vi "ge_HideCellCtrls.vi"(8 "error IO":errorcluster, 11 "FP Ctrl":T1) -> (0 "error out":errorcluster)   [LabVIEW 2018]
uses:
  Custom Ctrls/ge_FPCtrlRefLabel.ctl
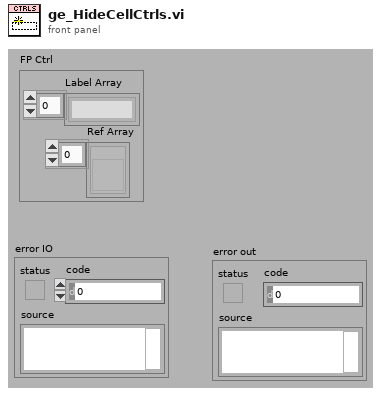
[diagram p1: front panel]
types:
  T1 = typedef "ge_FPCtrlRefLabel.ctl" = cluster{"Label Array":string[], "Ref Array":refnum<vi>[]}
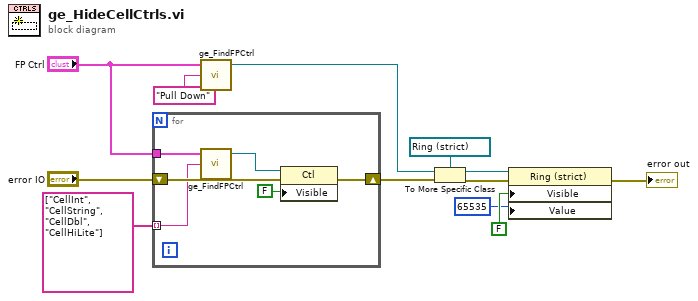
[diagram p0: block diagram]
diagram:
  n1 = for {
    shift-right: [w16] -> w8
    shift-left: "error IO" -> [w18]
    tunnel: string[] ["CellInt", "CellString", "CellDbl", "CellHiLite"] -> [w15] mode=indexing
    tunnel: "FP Ctrl" -> [w14]
    n2 = call "ge_FindFPCtrl.vi"("Ctrl Name"=w15, "FP Ctrl"=w14) -> ("Ctrl Ref"=w13:refnum<vi>)  [unwired: 3 in]
    n3 = property on="Property Node" class="Ctl"(reference=w13, error in=w18, "Visible"=FALSE) -> (error out=w16:errorcluster)  [unwired: 1 out]
  }
  n4 = call "ge_FindFPCtrl.vi"("Ctrl Name"="Pull Down" ("Name"), "FP Ctrl"="FP Ctrl") -> ("Ctrl Ref"=w5:refnum<vi>)  [unwired: 3 in]
  n5 = To More Specific Class(target class=refnum<vi> refnum ("reference"), reference=w5, error in=w8) -> (specific class reference=w1:refnum<vi>, error out=w4:errorcluster)
  n6 = property on="Property Node" class="Ring (strict)"(reference=w1, error in=w4, "Visible"=FALSE, "Value"=u16 65535) -> (error out=→"error out":errorcluster)  [unwired: 1 out]
